vi "Radoslaw_Wolnik_3.3.vi"() -> ()   [LabVIEW 2020]
panel:
  out "Ci¹g fibonacciego do 10 elementu":string
  # "Program oblicza 10 pierwszych wyrazów ci¹gu fibonacciego"
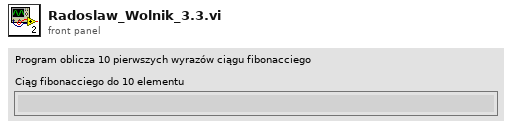
[diagram p1: front panel]
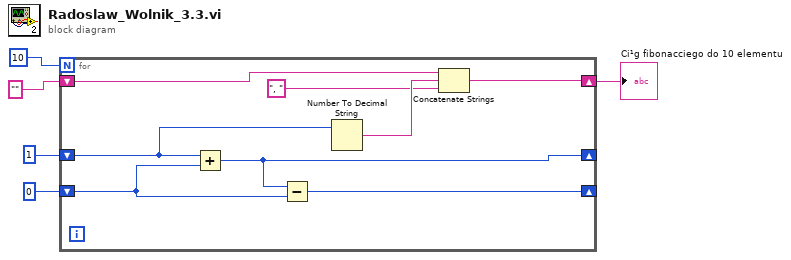
[diagram p0: block diagram]
diagram:
  n1 = for {
    N: 10 -> [_]
    shift-right: [w13] -> _
    shift-left: 0 -> [w10]
    shift-right: [w9] -> _
    shift-left: 1 -> [w8]
    shift-right: [w11] -> w3
    shift-left: "" -> [w12]
    n2 = Add(x=w8, y=w10) -> (x+y=w9:i32)
    n3 = Subtract(x=w9, y=w10) -> (x-y=w13:i32)
    n4 = Number To Decimal String(number=w8) -> (decimal integer string=w7:string)  [unwired: 1 in]
    n5 = Concatenate Strings(w12, w7, ", ") -> (w11:string)
  }
  "Ci¹g fibonacciego do 10 elementu" <- w3
